vi "Potting Data from Inspect Modules.vi"() -> ()   [LabVIEW 2011]
uses:
  Procedure Classes/Potting Procedure/Type Definitions/Inspect Modules - Module.ctl
  Shared Components/Vec3d Class/Vec3d Class.lvclass
  Shared Components/Utils/Type Definitions/Multi-Fiducial Image.ctl
  Shared Components/Utils/Type Definitions/Physical Image.ctl
  <vilib>/vision/Image Controls.llb/IMAQ Image.ctl
  Shared Components/Utils/Type Definitions/Fiducial with Source.ctl
  Shared Components/Utils/Type Definitions/Fiducial Image.ctl
  Shared Components/SyringeTool Class/Type Definitions/Module Potting Data.ctl
  Shared Components/Utils/Type Definitions/3d Line.ctl
panel:
  out "Module Potting Data":T1
  out "error out":errorcluster
  in  "error in":errorcluster
  in  "Module Data":T3={"TBM-TBM"={"Fiducial Image"={"Image Position"=refnum, "Image Reference"=refnum, "Field of View"={"x(mm)"=0.0, "y(mm)"=0.0}}, "Fiducials"=[]}, "TBM-HDI"={"Fiducial Image"={"Image Position"=refnum, "Image Reference"=refnum, "Field of View"={"x(mm)"=0.0, "y(mm)"=0.0}}, "Fiducials"=[]}, "Address Pads"={"Fiducial Image"={"Image Position"=refnum, "Image Reference"=refnum, "Field of View"={"x(mm)"=0.0, "y(mm)"=0.0}}, "Fiducials"=[]}, "HDI Bond Pad References"=[], "BBM Bond Pad References"=[], "HV-HDI"={"Fiducial Image"={"Image Position"=refnum, "Image Reference"=refnum, "Field of View"={"x(mm)"=0.0, "y(mm)"=0.0}}, "Selected Fiducial"={"Fiducial Image Coordinate"=refnum, "Fiducial Source"=enum."Pattern Recognition"}, "fiducial name"=""}, "HV-BBM"={"Fiducial Image"={"Image Position"=refnum, "Image Reference"=refnum, "Field of View"={"x(mm)"=0.0, "y(mm)"=0.0}}, "Selected Fiducial"={"Fiducial Image Coordinate"=refnum, "Fiducial Source"=enum."Pattern Recognition"}, "fiducial name"=""}, "Chuck"=0, "Slot"=0, "Potting Selection"={"HDI Bond Pads"=[TRUE, TRUE, TRUE, TRUE, TRUE, TRUE, TRUE, TRUE, TRUE, TRUE, TRUE, TRUE, TRUE, TRUE, TRUE, TRUE], "BBM Bond Pads"=[TRUE, TRUE, TRUE, TRUE, TRUE, TRUE, TRUE, TRUE, TRUE, TRUE, TRUE, TRUE, TRUE, TRUE, TRUE, TRUE], "TBM Inner"={"Top"=TRUE, "Left"=TRUE, "Bottom"=TRUE, "Right"=TRUE}, "TBM Outer"={"Top"=TRUE, "Left"=TRUE, "Bottom"=TRUE, "Right"=TRUE}, "Address Pads"={"Top"=TRUE, "Bottom"=TRUE}, "High Voltage"={"HDI"=TRUE, "Sensor"=TRUE}}}
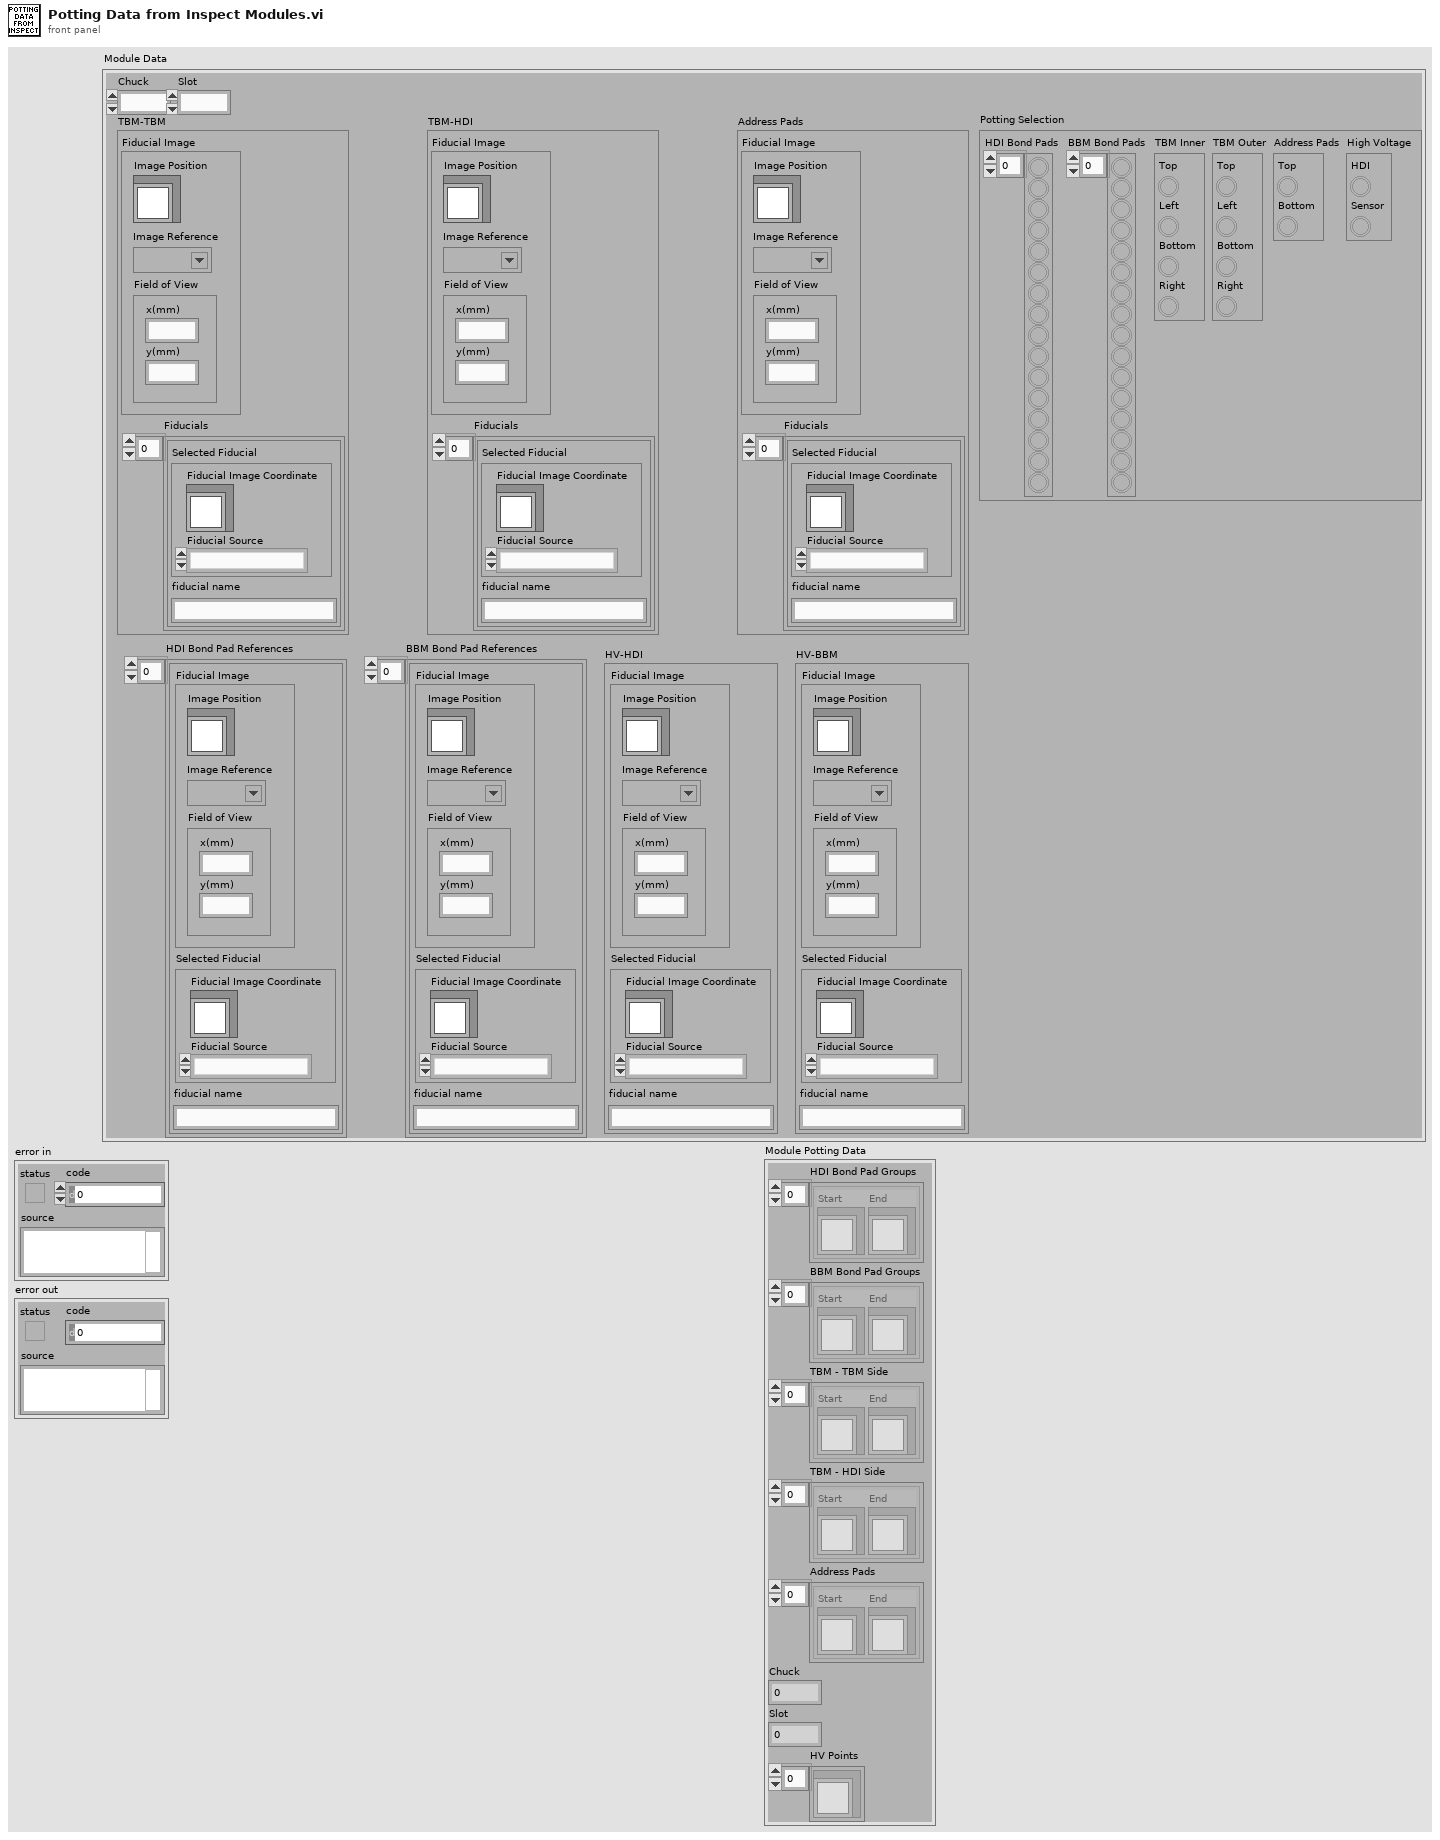
[diagram p1: front panel]
types:
  T1 = typedef "Module Potting Data.ctl" = cluster{"HDI Bond Pad Groups":T2[], "BBM Bond Pad Groups":T2[], "TBM - TBM Side":T2[], "TBM - HDI Side":T2[], "Address Pads":T2[], "Chuck":i32, "Slot":i32, "HV Points":refnum<class "Vec3d Class.lvclass">[]}
  T2 = typedef "3d Line.ctl" = cluster{"Start":refnum<class "Vec3d Class.lvclass">, "End":refnum<class "Vec3d Class.lvclass">}
  T3 = typedef "Inspect Modules - Module.ctl" = cluster{"TBM-TBM":T4, "TBM-HDI":T4, "Address Pads":T4, "HDI Bond Pad References":T8[], "BBM Bond Pad References":T8[], "HV-HDI":T8, "HV-BBM":T8, "Chuck":i32, "Slot":i32, "Potting Selection":cluster{"HDI Bond Pads":bool[], "BBM Bond Pads":bool[], "TBM Inner":cluster{"Top":bool, "Left":bool, "Bottom":bool, "Right":bool}, "TBM Outer":cluster{"Top":bool, "Left":bool, "Bottom":bool, "Right":bool}, "Address Pads":cluster{"Top":bool, "Bottom":bool}, "High Voltage":cluster{"HDI":bool, "Sensor":bool}}}
  T4 = typedef "Multi-Fiducial Image.ctl" = cluster{"Fiducial Image":T5, "Fiducials":cluster{"Selected Fiducial":T7, "fiducial name":string}[]}
  T5 = typedef "Physical Image.ctl" = cluster{"Image Position":refnum<class "Vec3d Class.lvclass">, "Image Reference":T6, "Field of View":cluster{"x(mm)":dbl, "y(mm)":dbl}}
  T6 = typedef "IMAQ Image.ctl" = refnum<image>
  T7 = typedef "Fiducial with Source.ctl" = cluster{"Fiducial Image Coordinate":refnum<class "Vec3d Class.lvclass">, "Fiducial Source":enum16{"Pattern Recognition", "User", "Error", "Default"}}
  T8 = typedef "Fiducial Image.ctl" = cluster{"Fiducial Image":T5, "Selected Fiducial":T7, "fiducial name":string}
  T9 = cluster{"Top":bool, "Left":bool, "Bottom":bool, "Right":bool}
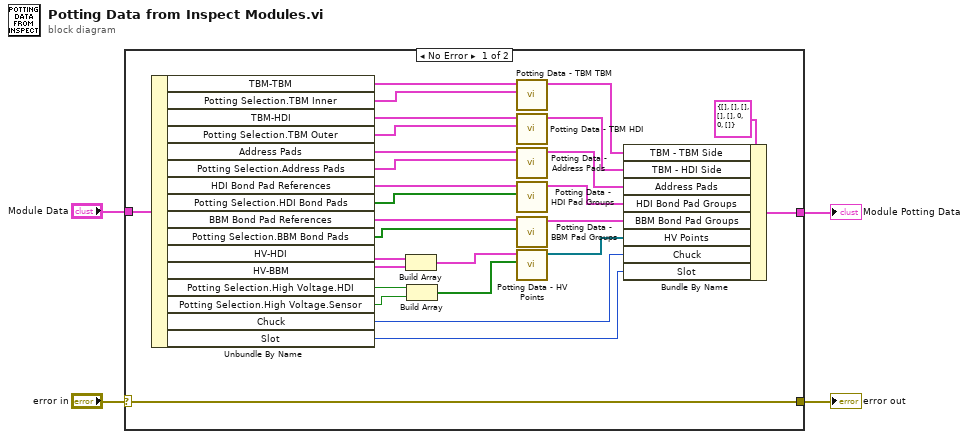
[diagram p0: block diagram]
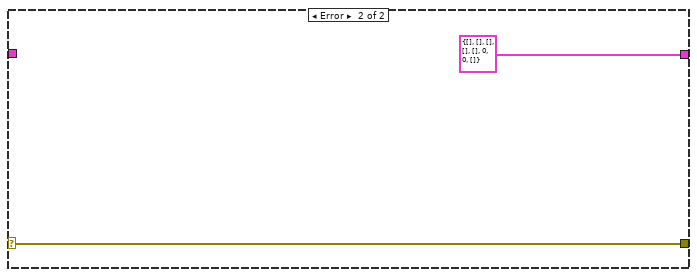
[diagram p2: hidden frame]
diagram:
  n1 = case shown="No Error" "error in" {
    selector: "error in" -> [w25 w34]
    tunnel: "Module Data" -> [w32 _]
    tunnel: [w25 w34] -> w2
    tunnel: [w5 T1 {"HDI Bond Pad Groups"=[], "BBM Bond Pad Groups"=[], "TBM - TBM Side"=[], "TBM - HDI Side"=[], "Address Pads"=[], "Chuck"=0, "Slot"=0, "HV Points"=[]} ("Module Potting Data")] -> w1
    frame No Error {
      n2 = Unbundle By Name(w32) -> ("TBM-TBM"=w31:T4, "Potting Selection.TBM Inner"=w30:T9, "TBM-HDI"=w29:T4, "Potting Selection.TBM Outer"=w28:T9, "Address Pads"=w27:T4, "Potting Selection.Address Pads"=w26:cluster{"Top":bool, "Bottom":bool}, "HDI Bond Pad References"=w24:T8[], "Potting Selection.HDI Bond Pads"=w23:bool[], "BBM Bond Pad References"=w22:T8[], "Potting Selection.BBM Bond Pads"=w21:bool[], "HV-HDI"=w20:T8, "HV-BBM"=w19:T8, "Potting Selection.High Voltage.HDI"=w18:bool, "Potting Selection.High Voltage.Sensor"=w17:bool, "Chuck"=w7:i32, "Slot"=w6:i32)
      n3 = Build Array(w20, w19) -> (w15:T8[])
      n4 = Build Array(w18, w17) -> (w16:bool[])
      n5 = call "Potting Data - TBM TBM.vi"("TBM-TBM Selection"=w30, "TBM-TBM Data"=w31) -> ("Potting Lines"=w13:T2[])  [unwired: 9 in]
      n6 = call "Potting Data - TBM HDI.vi"("TBM-HDI Selection"=w28, "TBM-HDI Data"=w29) -> ("Potting Lines"=w12:T2[])  [unwired: 9 in]
      n7 = call "Potting Data - Address Pads.vi"("Address Pads Selection"=w26, "Address Pads Data"=w27) -> ("Potting Lines"=w11:T2[])  [unwired: 9 in]
      n8 = call "Potting Data - HDI Pad Groups.vi"("Potting Selection HDI Bond Pads"=w23, "HDI Bond Pad References"=w24) -> ("Potting Lines"=w10:T2[])  [unwired: 8 in, 1 out]
      n9 = call "Potting Data - BBM Pad Groups.vi"("Potting Selection BBM Bond Pads"=w21, "BBM Bond Pad References"=w22) -> ("Potting Lines"=w9:T2[])  [unwired: 8 in, 1 out]
      n10 = call "Potting Data - HV Points.vi"("HV Point Selection"=w16, "HV Point Data"=w15) -> ("HV Potting Points"=w8:refnum<class "Vec3d Class.lvclass">[])  [unwired: 9 in]
      n11 = Bundle By Name(cluster=T1 {"HDI Bond Pad Groups"=[], "BBM Bond Pad Groups"=[], "TBM - TBM Side"=[], "TBM - HDI Side"=[], "Address Pads"=[], "Chuck"=0, "Slot"=0, "HV Points"=[]} ("Module Potting Data"), "TBM - TBM Side"=w13, "TBM - HDI Side"=w12, "Address Pads"=w11, "HDI Bond Pad Groups"=w10, "BBM Bond Pad Groups"=w9, "HV Points"=w8, "Chuck"=w7, "Slot"=w6) -> (w5:T1)
    }
    frame Error {
    }
  }
  "error out" <- w2
  "Module Potting Data" <- w1
